vi "Obtain Last Clone Instance Notifier.vi"() -> (1 "created new?":bool, 3 "Last Instance Notifier":refnum<notifier>)   [LabVIEW 2020, in "Hardware Interface.lvlib" / "Clone Registration.lvlib"]
doc: "Obtains a named notifier that is fired whenever the last instance of a cloneable module is stopped.\n_____\nBased on Delacor QMH Project Template 5.0.0.82."
uses:
  Clone Registration.lvlib
  Hardware Interface.lvlib
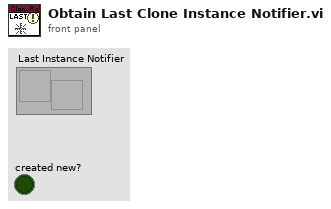
[diagram p1: front panel]
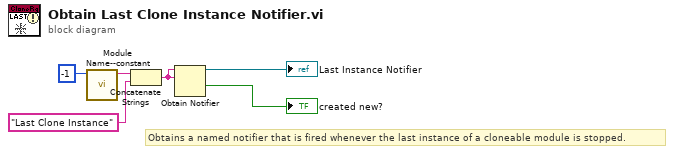
[diagram p0: block diagram]
diagram:
  # "Obtains a named notifier that is fired whenever the last instance of a cloneable module is stopped."
  n1 = call "Module Name--constant.vi"("Module ID"=-1) -> ("Module Name"=w3:string)  [unwired: 10 in]
  n2 = Concatenate Strings(w3, "Last Clone Instance" ("string")) -> (w4:string)
  n3 = Obtain Notifier(name (unnamed)=w4, notification data type=w4) -> (notifier out=→"Last Instance Notifier":refnum<notifier>, created new?=→"created new?":bool)  [unwired: 2 in, 1 out]
